vi "PCO_SetBitAlignmente.vi"(8 "error in (no error)":errorcluster, 10 "wBitAlignment":enum16{"MSB", "LSB"}(ring), 11 "Handle":u64) -> (0 "error out":errorcluster, 3 "Handle Out":u64, 5 "return type":u32 format="%x")   [LabVIEW 2011]
uses:
  SC2_Cam64.dll
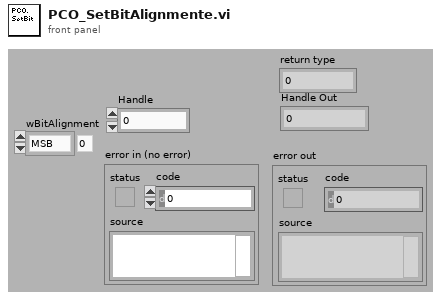
[diagram p1: front panel]
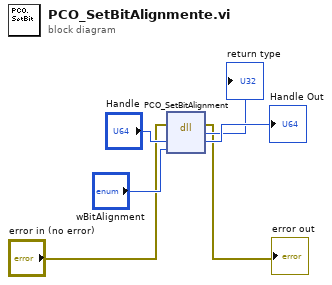
[diagram p0: block diagram]
diagram:
  n1 = dll-call lib="SC2_Cam*.*" fn="PCO_SetBitAlignment"(error in="error in (no error)", "Handle"="Handle", "wBitAlignment"="wBitAlignment") -> (error out=→"error out":errorcluster, "return type"=→"return type":u64, "Handle"=→"Handle Out":u64)  [unwired: 2 in, 2 out]
